vi "Count Receivers.vi"(8 "error in (no error)":errorcluster, 11 "Pub Sub Message Channel in":refnum<class "Pub Sub Message Channel.lvclass">) -> (0 "error out":errorcluster, 2 "size":i32, 3 "Pub Sub Message Channel out":refnum<class "Pub Sub Message Channel.lvclass">)   [LabVIEW 2020, in "Actor Pub Sub Channels.lvlib" / "Pub Sub Message Channel.lvclass"]
uses:
  Pub Sub Message Channel.lvclass
  Pub Sub Message Channel.lvclass/Pub Sub Message Channel.ctl
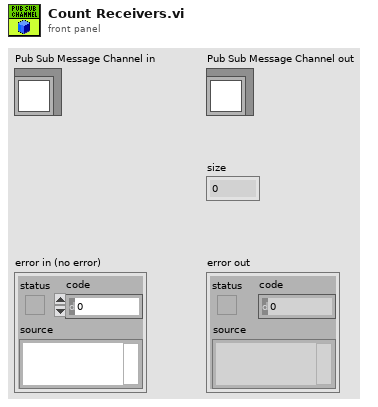
[diagram p1: front panel]
types:
  T1 = map{refnum<class "Message Enqueuer.lvclass">, cluster{"Name":string, "Included (All)":refnum<class "Message.lvclass">[], "Excluded (None)":refnum<class "Message.lvclass">[]}}
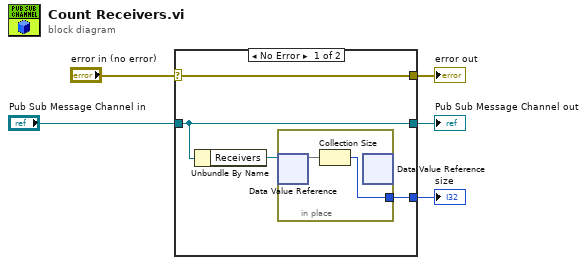
[diagram p0: block diagram]
diagram:
  n1 = case shown="No Error" "error in (no error)" {
    selector: "error in (no error)" -> [w9 w13]
    tunnel: [w9 w13] -> w4
    tunnel: [w8 w12] -> w2
    tunnel: "Pub Sub Message Channel in" -> [w8 w12]
    tunnel: [w6 _] -> w1
    frame No Error {
      n2 = Unbundle By Name(w8) -> ("Receivers"=w7:refnum<data-value>)
      n3 = in-place {
        in-place-border: [w10] -> w6
        n4 = in-place-dvr #1(w7) -> (w11:T1)  [unwired: 1 out]
        n5 = Collection Size(1:w11) -> (0:w10:i32)
        n6 = in-place-dvr #1() -> ()  [unwired: 1 in, 2 out]
      }
    }
    frame Error {
    }
  }
  "error out" <- w4
  "Pub Sub Message Channel out" <- w2
  "size" <- w1
